vi "StarImg-Dark.vi"(1 "Tableau":i32[][](array[numeric])) -> (0 "Intensité":sgl format="%.2f")   [LabVIEW 2011]
panel:
  out "Sous-total":i32
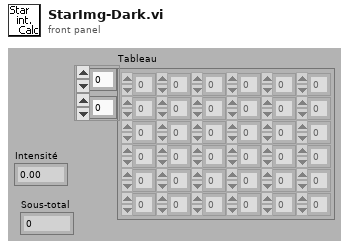
[diagram p1: front panel]
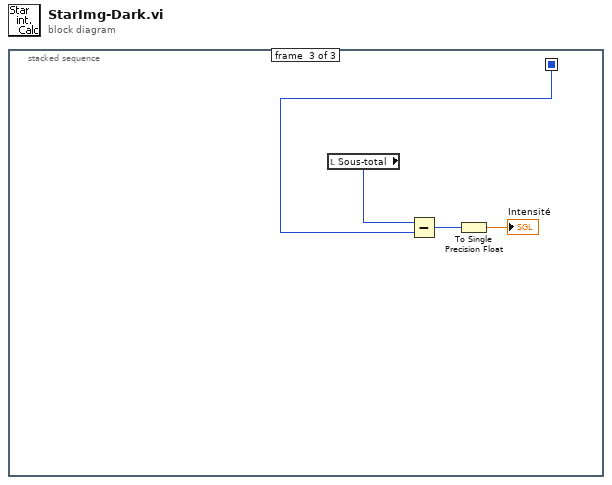
[diagram p0: block diagram]
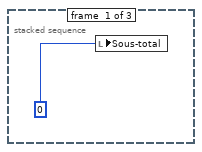
[diagram p2: hidden frame]
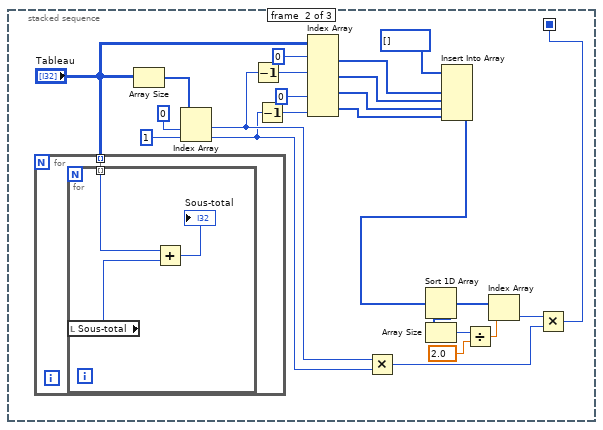
[diagram p3: hidden frame]
diagram:
  n1 = stacked-sequence {
    seq-local: [_ w18 _] -> [_ _ w30]
    frame #0 {
      n2 = local write "Sous-total"(0) -> ()
    }
    frame #1 {
      n3 = for {
        tunnel: "Tableau" -> [w25] mode=indexing
        n4 = for {
          tunnel: w25 -> [w28] mode=indexing
          n5 = local read "Sous-total"() -> (w26:i32)
          n6 = Add(x=w28, y=w26) -> (x+y=→"Sous-total":i32)
        }
      }
      n7 = Array Size(array="Tableau") -> (size(s)=w23:i32[])
      n8 = Index Array(array=w23, index #1=0 ("indice"), index #2=1 ("indice")) -> (element #1=w10:i32, element #2=w9:i32)
      n9 = Decrement(x=w10) -> (x-1=w17:i32)
      n10 = Decrement(x=w9) -> (x-1=w16:i32)
      n11 = Index Array(array="Tableau", index (row) #1=0 ("indice (ligne)"), index (row) #2=w17, index (col) #3=0 ("indice (ligne)"), index (col) #4=w16) -> (element #1=w7:i32[], element #2=w6:i32[], element #3=w5:i32[], element #4=w4:i32[])  [unwired: 4 in]
      n12 = Multiply(x=w10, y=w9) -> (x*y=w2:i32)
      n13 = Insert Into Array(array=i32[] [] ("tableau"), new element #1=w7, new element #2=w6, new element #3=w5, new element #4=w4) -> (w3:i32[])  [unwired: 1 in]
      n14 = Sort 1D Array(array=w3) -> (sorted array=w15:i32[])
      n15 = Array Size(array=w15) -> (size(s)=w14:i32)
      n16 = Divide(x=w14, y=2.0) -> (x/y=w12:dbl)
      n17 = Index Array(array=w15, index=w12) -> (element=w11:i32)
      n18 = Multiply(x=w11, y=w2) -> (x*y=w18:i32)
    }
    frame #2 {
      n19 = local read "Sous-total"() -> (w31:i32)
      n20 = Subtract(x=w31, y=w30) -> (x-y=w32:i32)
      n21 = To Single Precision Float(number=w32) -> (single precision float=→"Intensité":sgl)
    }
  }
